vi "Host-FPGA Interface.vi"(6 "error in":errorcluster, 8 "Interface":T2, 9 "Dynamic Ref In":T1) -> (0 "error out":errorcluster, 1 "Recording":bool, 3 "Dynamic Ref Out":T1)   [LabVIEW 2015]
uses:
  TypeDefs Host/Interface Items.ctl
  TypeDefs Host/FPGA Dynamic Interface.ctl
  <vilib>/Utility/error.llb/Error Cluster From Error Code.vi
  <vilib>/rvi/errors/niLvFpgaAdjustHostInterfaceError.vi
  <vilib>/rvi/interface/nirviReadWriteControl/nirviReadWriteControl.xnode
  NiFpgaLv.dll
  <vilib>/rvi/interface/Simulation/niFpgaSimulationCallBeginRW.vi
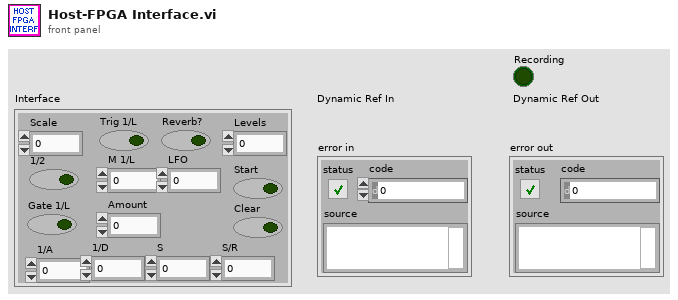
[diagram p1: front panel]
types:
  T1 = typedef "FPGA Dynamic Interface.ctl" = refnum<k20>
  T2 = typedef "Interface Items.ctl" = cluster{"Scale":u8, "Trig 1/L":bool, "Start":bool, "Clear":bool, "Reverb?":bool, "Levels":u8, "M 1/L":fxp<+,32,32>, "Gate 1/L":bool, "LFO":fxp<+/-,8,8>, "Amount":fxp<+,8,0>, "1/A":fxp<+,16,0>, "1/D":fxp<+,16,0>, "S":fxp<+,16,0>, "S/R":fxp<+,16,0>, "1/2":bool}
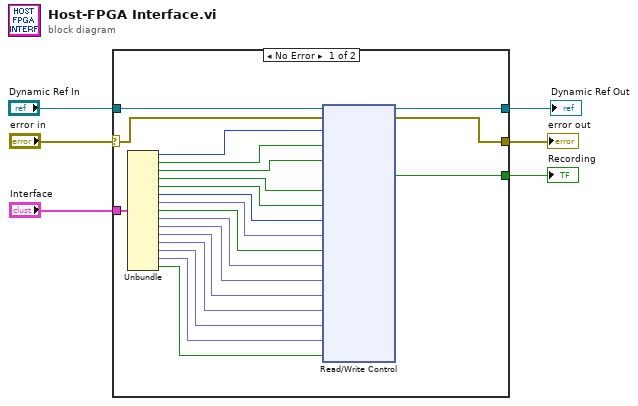
[diagram p0: block diagram]
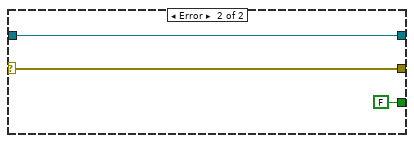
[diagram p2: hidden frame]
diagram:
  n1 = case shown="No Error" "error in" {
    selector: "error in" -> [w25 w29]
    tunnel: [w27 w30] -> w1
    tunnel: "Dynamic Ref In" -> [w26 w30]
    tunnel: "Interface" -> [w22 _]
    tunnel: [w24 w29] -> w4
    tunnel: [w23 FALSE ("Recording")] -> w3
    frame No Error {
      n2 = Unbundle(w22) -> ("Scale"=w21:u8, "Trig 1/L"=w20:bool, "Start"=w19:bool, "Clear"=w18:bool, "Reverb?"=w17:bool, "Levels"=w16:u8, "M 1/L"=w15:fxp<+,32,32>, "Gate 1/L"=w14:bool, "LFO"=w13:fxp<+/-,8,8>, "Amount"=w12:fxp<+,8,0>, "1/A"=w11:fxp<+,16,0>, "1/D"=w10:fxp<+,16,0>, "S"=w9:fxp<+,16,0>, "S/R"=w8:fxp<+,16,0>, "1/2"=w7:bool)
      n3 = xnode "Read/Write Control"("FPGA VI Reference In"=w26, "error in"=w25, "Scale"=w21, "Trigger"=w20, "Start"=w19, "Clear?"=w18, "Delay?"=w17, "Levels"=w16, "M"=w15, "Gate"=w14, "LFO"=w13, "Amount"=w12, "1/Attack"=w11, "1/Decay"=w10, "Sustain"=w9, "S/R"=w8, "1/2"=w7) -> ("FPGA VI Reference Out"=w27:T1, "error out"=w24:errorcluster, "Recording"=w23:bool)
    }
    frame Error {
    }
  }
  "error out" <- w4
  "Recording" <- w3
  "Dynamic Ref Out" <- w1
